vi "Connect with Connection File.vi"(8 "error in (no error)":errorcluster, 10 "Connection File (default=guess)":path, 11 "object in":refnum<class "JuPyter_Client.lvclass">) -> (0 "error out":errorcluster, 3 "object out":refnum<class "JuPyter_Client.lvclass">)   [LabVIEW 2018, in "JuPyter_Client.lvclass"]
doc: "Connect to an existing kernel"
uses:
  JuPyter_Client.lvclass
  JuPyter_Client.lvclass/JuPyter_Client.ctl
  <vilib>/addons/zeromq/socket_type.ctl
  <vilib>/addons/zeromq/socket_options.ctl
  <vilib>/addons/zeromq/zmq_socket.lvclass
  ClientMessaging.lvlib
  <vilib>/addons/zeromq/zmq_context.lvclass
  <vilib>/addons/zeromq/zeromq.lvlib
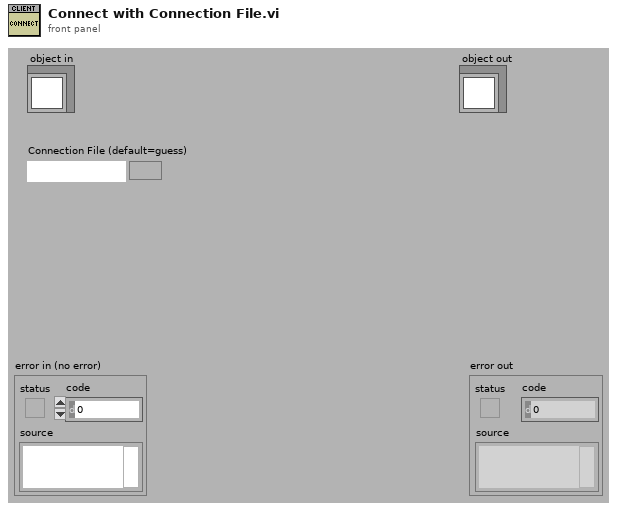
[diagram p1: front panel]
types:
  T1 = enum16{"Shell", "IOPub", "Stdin", "Control", "Heart Beat"}
  T2 = typedef "zeromq.lvlib/socket_type.ctl" = enum8{"ZMQ_PAIR", "ZMQ_PUB", "ZMQ_SUB", "ZMQ_REQ", "ZMQ_REP", "ZMQ_DEALER", "ZMQ_ROUTER", "ZMQ_PULL", "ZMQ_PUSH", "ZMQ_XPUB", "ZMQ_XSUB"}
  T3 = typedef "zeromq.lvlib/socket_options.ctl" = enum8{"NONE", "ZMQ_HWM", "<2>", "ZMQ_SWAP", "ZMQ_AFFINITY", "ZMQ_IDENTITY", "ZMQ_SUBSCRIBE", "ZMQ_UNSUBSCRIBE", "ZMQ_RATE", "ZMQ_RECOVERY_IVL", "ZMQ_MCAST_LOOP", "ZMQ_SNDBUF", "ZMQ_RCVBUF", "ZMQ_RCVMORE", "ZMQ_FD", "ZMQ_EVENTS", "ZMQ_TYPE", "ZMQ_LINGER", "ZMQ_RECONNECT_IVL", "ZMQ_BACKLOG", "ZMQ_RECOVERY_IVL_MSEC", "ZMQ_RECONNECT_IVL_MAX", "ZMQ_MAXMSGSIZE", "ZMQ_SNDHWM", "ZMQ_RCVHWM", "ZMQ_MULTICAST_HOPS", "<26>", "ZMQ_RCVTIMEO", "ZMQ_SNDTIMEO", "<29>", "<30>", "ZMQ_IPV4ONLY", "ZMQ_LAST_ENDPOINT", "ZMQ_ROUTER_MANDATORY", "ZMQ_TCP_KEEPALIVE", "ZMQ_TCP_KEEPALIVE_CNT", "ZMQ_TCP_KEEPALIVE_IDLE", "ZMQ_TCP_KEEPALIVE_INTVL", "ZMQ_TCP_ACCEPT_FILTER", "ZMQ_DELAY_ATTACH_ON_CONNECT", "ZMQ_XPUB_VERBOSE"}
  T4 = typedef "ClientMessaging.lvlib/Connection.ctl" = cluster{"transport":string, "ip":string, "key":string, "signature_scheme":string, "kernel_name":string, "shell_port":u16, "iopub_port":u16, "stdin_port":u16, "control_port":u16, "hb_port":u16}
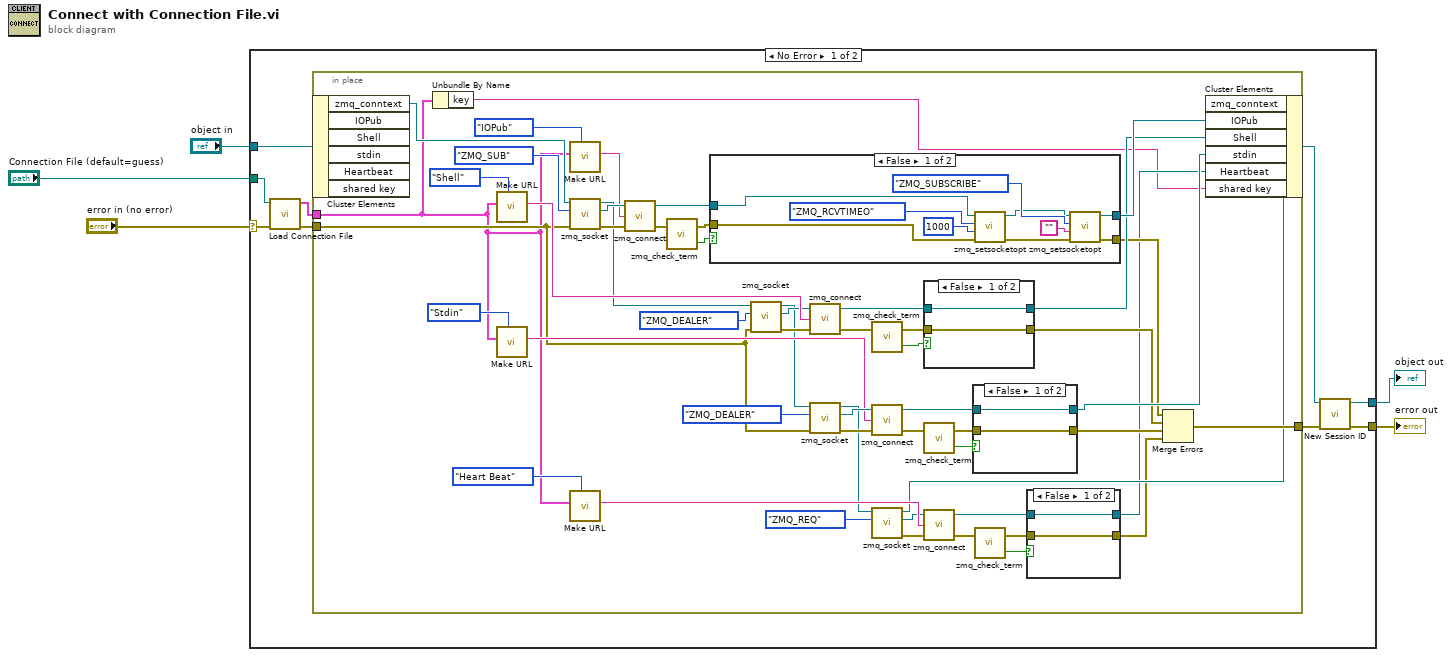
[diagram p0: block diagram]
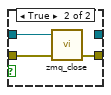
[diagram p2: hidden frame]
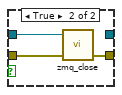
[diagram p3: hidden frame]
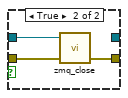
[diagram p4: hidden frame]
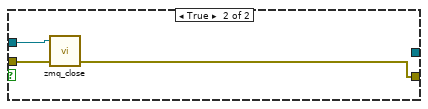
[diagram p5: hidden frame]
diagram:
  n1 = case shown="No Error" "error in (no error)" {
    selector: "error in (no error)" -> [w9 w97]
    tunnel: [w6 w97] -> w4
    tunnel: [w8 w96] -> w2
    tunnel: "object in" -> [w13 w96]
    tunnel: "Connection File (default=guess)" -> [w14 _]
    frame No Error {
      n2 = call "Load Connection File.vi"("error in (no error)"=w9, "Path to Connection File"=w14) -> ("error out"=w11:errorcluster, "Connection Info"=w12:T4)  [unwired: 8 in]
      n3 = in-place {
        in-place-border: w12 -> [w16]
        in-place-border: w11 -> [w36]
        in-place-border: [w30] -> w7
        n4 = in-place-cluster #1(w13) -> ("zmq_conntext"=w67:refnum<class "zmq_context.lvclass">)  [unwired: 5 out]
        n5 = Unbundle By Name(w16) -> ("key"=w15:string)
        n6 = call "Make URL.vi"("Port"=T1."Shell", "Connection Info"=w16) -> ("Connection URL"=w52:string)  [unwired: 9 in]
        n7 = call "Make URL.vi"("Port"=T1."Stdin", "Connection Info"=w16) -> ("Connection URL"=w47:string)  [unwired: 9 in]
        n8 = call "Make URL.vi"("Port"=T1."IOPub", "Connection Info"=w16) -> ("Connection URL"=w64:string)  [unwired: 9 in]
        n9 = call <vilib>:"zmq_socket.vi"("error in"=w36, "socket type"=socket_type."ZMQ_SUB", "context in"=w67) -> ("error out"=w63:errorcluster, "socket out"=w65:refnum<class "zmq_socket.lvclass">, "context out"=w41:refnum<class "zmq_context.lvclass">)  [unwired: 2 in]
        n10 = call "Make URL.vi"("Port"=T1."Heart Beat", "Connection Info"=w16) -> ("Connection URL"=w23:string)  [unwired: 9 in]
        n11 = call <vilib>:"zmq_connect.vi"("error in"=w63, "endpoint"=w64, "socket in"=w65) -> ("error out"=w62:errorcluster, "socket out"=w60:refnum<class "zmq_socket.lvclass">)  [unwired: 1 in]
        n12 = call <vilib>:"zmq_check_term.vi"("error in"=w62) -> ("term?"=w61:bool, "error out"=w59:errorcluster)  [unwired: 1 in]
        n13 = case shown="False" w61 {
          tunnel: w60 -> [w87 w95]
          tunnel: w59 -> [w88 w94]
          tunnel: [w90 w93] -> w33
          tunnel: [w92 _] -> w58
          frame False {
            n14 = call <vilib>:"zmq_setsocketopt.vi"("error in"=w88, "value"=1000, "option"=socket_options."ZMQ_RCVTIMEO", "socket in"=w87) -> ("error out"=w86:errorcluster, "socket out"=w85:refnum<class "zmq_socket.lvclass">)  [unwired: 2 in]
            n15 = call <vilib>:"zmq_setsocketopt.vi"("error in"=w86, "value"="", "option"=socket_options."ZMQ_SUBSCRIBE", "socket in"=w85) -> ("error out"=w90:errorcluster, "socket out"=w92:refnum<class "zmq_socket.lvclass">)  [unwired: 2 in]
          }
          frame True {
            n16 = call <vilib>:"zmq_close.vi"("error in"=w94, "socket"=w95) -> ("error out"=w93:errorcluster)  [unwired: 3 in]
          }
        }
        n17 = call <vilib>:"zmq_socket.vi"("error in"=w36, "socket type"=socket_type."ZMQ_DEALER", "context in"=w41) -> ("error out"=w53:errorcluster, "socket out"=w51:refnum<class "zmq_socket.lvclass">, "context out"=w40:refnum<class "zmq_context.lvclass">)  [unwired: 2 in]
        n18 = call <vilib>:"zmq_connect.vi"("error in"=w53, "endpoint"=w52, "socket in"=w51) -> ("error out"=w54:errorcluster, "socket out"=w56:refnum<class "zmq_socket.lvclass">)  [unwired: 1 in]
        n19 = call <vilib>:"zmq_socket.vi"("error in"=w36, "socket type"=socket_type."ZMQ_DEALER", "context in"=w40) -> ("error out"=w46:errorcluster, "socket out"=w48:refnum<class "zmq_socket.lvclass">, "context out"=w20:refnum<class "zmq_context.lvclass">)  [unwired: 2 in]
        n20 = call <vilib>:"zmq_check_term.vi"("error in"=w54) -> ("term?"=w55:bool, "error out"=w57:errorcluster)  [unwired: 1 in]
        n21 = call <vilib>:"zmq_connect.vi"("error in"=w46, "endpoint"=w47, "socket in"=w48) -> ("error out"=w45:errorcluster, "socket out"=w43:refnum<class "zmq_socket.lvclass">)  [unwired: 1 in]
        n22 = call <vilib>:"zmq_socket.vi"("socket type"=socket_type."ZMQ_REQ", "context in"=w20) -> ("error out"=w24:errorcluster, "socket out"=w22:refnum<class "zmq_socket.lvclass">, "context out"=w19:refnum<class "zmq_context.lvclass">)  [unwired: 3 in]
        n23 = case shown="False" w55 {
          tunnel: w56 -> [w78 w82]
          tunnel: w57 -> [w79 w81]
          tunnel: [w79 w80] -> w32
          tunnel: [w78 _] -> w35
          frame False {
          }
          frame True {
            n24 = call <vilib>:"zmq_close.vi"("error in"=w81, "socket"=w82) -> ("error out"=w80:errorcluster)  [unwired: 3 in]
          }
        }
        n25 = call <vilib>:"zmq_check_term.vi"("error in"=w45) -> ("term?"=w44:bool, "error out"=w42:errorcluster)  [unwired: 1 in]
        n26 = call <vilib>:"zmq_connect.vi"("error in"=w24, "endpoint"=w23, "socket in"=w22) -> ("error out"=w25:errorcluster, "socket out"=w27:refnum<class "zmq_socket.lvclass">)  [unwired: 1 in]
        n27 = case shown="False" w44 {
          tunnel: w43 -> [w73 w77]
          tunnel: w42 -> [w74 w76]
          tunnel: [w74 w75] -> w31
          tunnel: [w73 _] -> w34
          frame False {
          }
          frame True {
            n28 = call <vilib>:"zmq_close.vi"("error in"=w76, "socket"=w77) -> ("error out"=w75:errorcluster)  [unwired: 3 in]
          }
        }
        n29 = call <vilib>:"zmq_check_term.vi"("error in"=w25) -> ("term?"=w26:bool, "error out"=w28:errorcluster)  [unwired: 1 in]
        n30 = case shown="False" w26 {
          tunnel: w27 -> [w68 w72]
          tunnel: w28 -> [w69 w71]
          tunnel: [w69 w70] -> w17
          tunnel: [w68 _] -> w18
          frame False {
          }
          frame True {
            n31 = call <vilib>:"zmq_close.vi"("error in"=w71, "socket"=w72) -> ("error out"=w70:errorcluster)  [unwired: 3 in]
          }
        }
        n32 = Merge Errors(w33, w32, w31, w17) -> (w30:errorcluster)
        n33 = in-place-cluster #1("zmq_conntext"=w19, "IOPub"=w58, "Shell"=w35, "stdin"=w34, "Heartbeat"=w18, "shared key"=w15) -> (w10:refnum<class "JuPyter_Client.lvclass">)
      }
      n34 = call-dynamic "New Session ID.vi"("error in (no error)"=w7, "object in"=w10) -> ("error out"=w6:errorcluster, "object out"=w8:refnum<class "JuPyter_Client.lvclass">)  [unwired: 8 in]
    }
    frame Error {
    }
  }
  "error out" <- w4
  "object out" <- w2
